vi "Read Logger.vi"(8 "error in (no error)":errorcluster, 11 "Log Word Message in":refnum<class "Log Word Message.lvclass">) -> (0 "error out":errorcluster, 2 "Logger":T1, 3 "Log Word Message out":refnum<class "Log Word Message.lvclass">)   [LabVIEW 2020, in "Ballard ARINC 429 Engine.lvlib" / "Implementation.lvlib" / "Word Logging.lvlib" / "Log Word Message.lvclass"]
uses:
  Log Word Message.lvclass
  Log Word Message.lvclass/Log Word Message.ctl
  Word Logger Interface/Word Logger Interface.lvclass
  Word Logger Data Reference.ctl
  Word Logging.lvlib
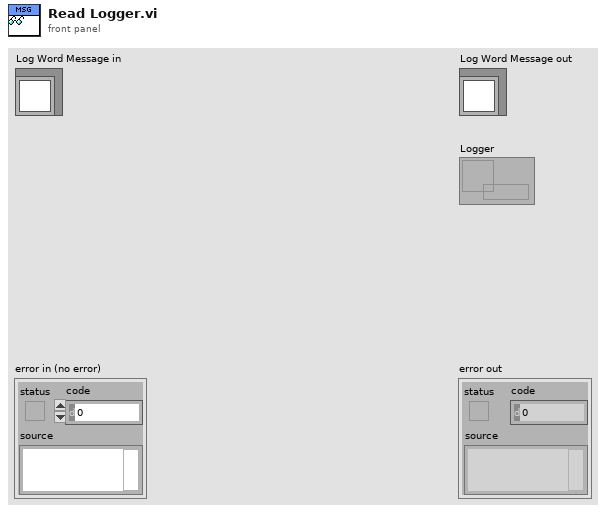
[diagram p1: front panel]
types:
  T1 = typedef "Ballard ARINC 429 Engine.lvlib/Implementation.lvlib/Word Logging.lvlib/Word Logger Data Reference.ctl" = refnum<data-value>
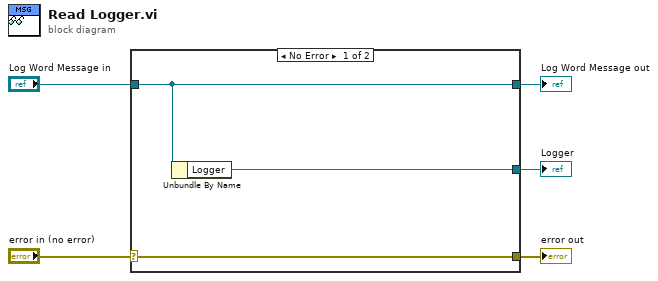
[diagram p0: block diagram]
diagram:
  n1 = case shown="No Error" "error in (no error)" {
    selector: "error in (no error)" -> [w8 w9]
    tunnel: [w8 w9] -> w4
    tunnel: [w7 w10] -> w2
    tunnel: "Log Word Message in" -> [w7 w10]
    tunnel: [w6 _] -> w1
    frame No Error {
      n2 = Unbundle By Name(w7) -> ("Logger"=w6:T1)
    }
    frame Error {
    }
  }
  "error out" <- w4
  "Log Word Message out" <- w2
  "Logger" <- w1
